vi "stop_message.vi"(9 "识别符":string, 10 "notifier":refnum<notifier>) -> (1 "通知":string, 3 "Exit？":bool)   [LabVIEW 2012]
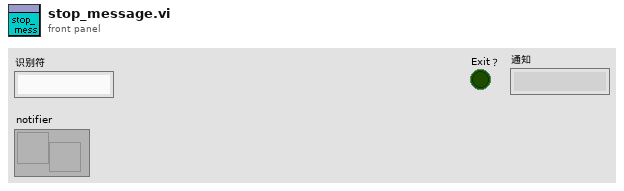
[diagram p1: front panel]
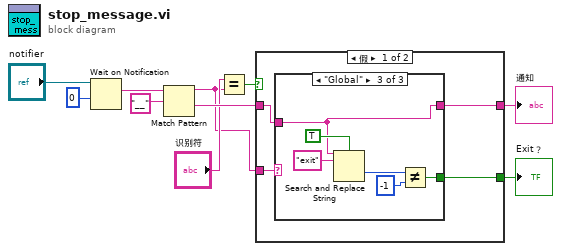
[diagram p0: block diagram]
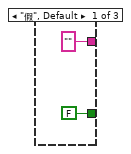
[diagram p2: hidden frame]
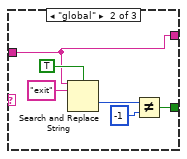
[diagram p3: hidden frame]
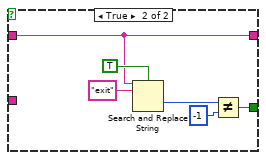
[diagram p4: hidden frame]
diagram:
  n1 = Wait on Notification(notifier="notifier", timeout in ms (-1)=0 ("超时毫秒(-1)")) -> (notification=w8:string)  [unwired: 2 in, 3 out]
  n2 = Match Pattern(string=w8, regular expression="__" ("正则表达式")) -> (before substring=w3:string, after substring=w9:string)  [unwired: 1 in, 2 out]
  n3 = Equal?(x="识别符", y=w3) -> (x = y?=w6:bool)
  n4 = case shown="假" w6 {
    tunnel: [w13 w30] -> w10
    tunnel: w9 -> [w11 w29]
    tunnel: [w14 w29] -> w5
    tunnel: w3 -> [w12 _]
    frame False {
      n5 = case shown="\"Global\"" w12 {
        tunnel: ["" w17 w23] -> w14
        tunnel: [FALSE w18 w24] -> w13
        tunnel: w11 -> [_ w17 w23]
        frame "假", Default {
        }
        frame "global" {
          n6 = Search and Replace String(case sensitive?=TRUE ("忽略大小写？(F)"), input string=w17, search string="exit" ("搜索字符串")) -> (offset past replacement=w20:i32)  [unwired: 5 in, 3 out]
          n7 = Not Equal?(x=w20, y=-1) -> (x != y?=w18:bool)
        }
        frame "Global" {
          n8 = Search and Replace String(case sensitive?=TRUE ("忽略大小写？(F)"), input string=w23, search string="exit" ("搜索字符串")) -> (offset past replacement=w26:i32)  [unwired: 5 in, 3 out]
          n9 = Not Equal?(x=w26, y=-1) -> (x != y?=w24:bool)
        }
      }
    }
    frame True {
      n10 = Search and Replace String(case sensitive?=TRUE ("忽略大小写？(F)"), input string=w29, search string="exit" ("搜索字符串")) -> (offset past replacement=w32:i32)  [unwired: 5 in, 3 out]
      n11 = Not Equal?(x=w32, y=-1) -> (x != y?=w30:bool)
    }
  }
  "Exit？" <- w10
  "通知" <- w5
